vi "Convert Format to Resource Type.vi"(10 "Use VTT?":bool) -> (1 "BD Resource Type":string, 2 "FP Resource Type":string, 3 "Heap Save Format":T1=1 items=["Off", "XML", "Binary", "Verbose Tagged Text", "Binary2"])   [LabVIEW 2023]
uses:
  Resource Manipulation/Heap Save Format.ctl
  Resource Manipulation.lvlib
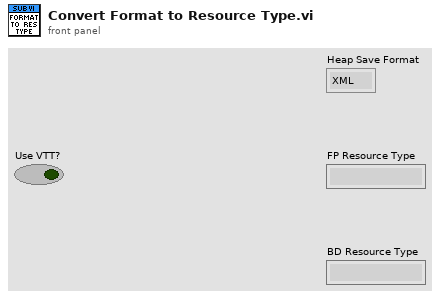
[diagram p1: front panel]
types:
  T1 = typedef "Resource Manipulation.lvlib/Heap Save Format.ctl" = u16
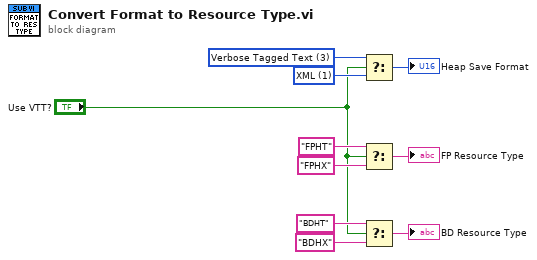
[diagram p0: block diagram]
diagram:
  w6 = T1 3 items=["Off", "XML", "Binary", "Verbose Tagged Text", "Binary2"] ("Heap Save Format (1=XML)")
  w5 = T1 1 items=["Off", "XML", "Binary", "Verbose Tagged Text", "Binary2"] ("Heap Save Format (1=XML)")
  n1 = Select(t=w6, s="Use VTT?", f=w5) -> (s? t:f=→"Heap Save Format":T1)
  n2 = Select(t="FPHT", s="Use VTT?", f="FPHX") -> (s? t:f=→"FP Resource Type":string)
  n3 = Select(t="BDHT", s="Use VTT?", f="BDHX") -> (s? t:f=→"BD Resource Type":string)
